vi "Split Version.vi"(11 "VI Version":string) -> (0 "Current Revision":u32, 1 "Current Phase":T1, 2 "Minor Version":u16, 3 "Major Version":u16)   [LabVIEW 2014]
uses:
  TYPE_Version Status.ctl
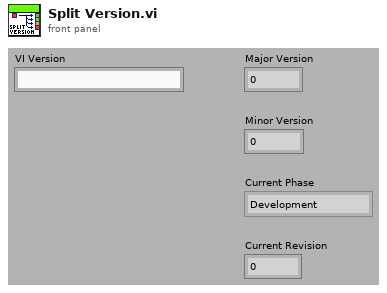
[diagram p1: front panel]
types:
  T1 = typedef "TYPE_Version Status.ctl" = enum16{"Development", "alpha", "beta", "Reviewed", "Bug", "Other"}
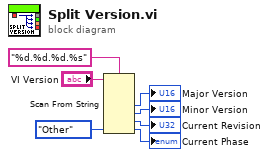
[diagram p0: block diagram]
diagram:
  n1 = Scan From String(format string="%d.%d.%d.%s" ("Author"), input string="VI Version", default 4=TYPE_Version_Status."Other" ("Current Phase")) -> (output 1=→"Major Version":u16, output 2=→"Minor Version":u16, output 3=→"Current Revision":u32, output 4=→"Current Phase":T1)  [unwired: 5 in, 3 out]
